vi "Write Diagram.vi"(8 "error in (no error)":errorcluster, 10 "Diagram":refnum<vi>, 11 "Structures in":refnum<class "Structures.lvclass">) -> (0 "error out":errorcluster, 3 "Structures out":refnum<class "Structures.lvclass">)   [LabVIEW 2015, in "Structures.lvclass"]
uses:
  Structures.lvclass
  Structures.lvclass/Structures.ctl
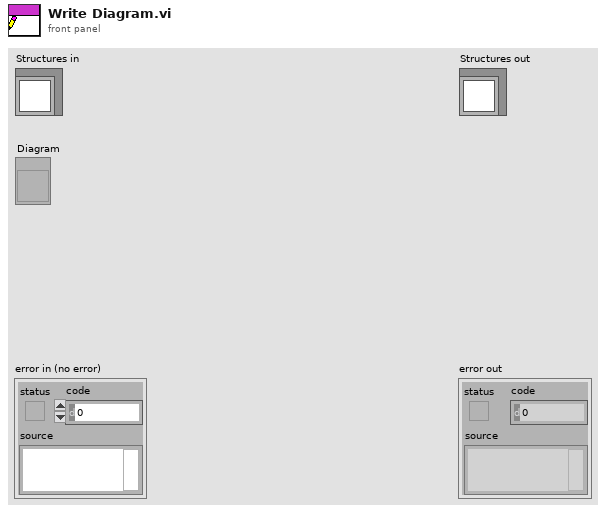
[diagram p1: front panel]
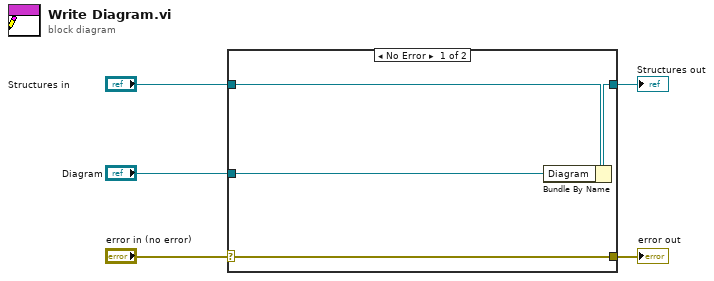
[diagram p0: block diagram]
diagram:
  n1 = case shown="No Error" "error in (no error)" {
    selector: "error in (no error)" -> [w9 w10]
    tunnel: [w9 w10] -> w4
    tunnel: [w7 w11] -> w2
    tunnel: "Structures in" -> [w8 w11]
    tunnel: "Diagram" -> [w6 _]
    frame No Error {
      n2 = Bundle By Name(cluster=w8, "Diagram"=w6) -> (w7:refnum<class "Structures.lvclass">)
    }
    frame Error {
    }
  }
  "error out" <- w4
  "Structures out" <- w2
